vi "SendNoReply.vi"(8 "error in (no error)":errorcluster, 10 "DataIn":string, 11 "index":i32) -> (0 "error out":errorcluster)   [LabVIEW 2019]
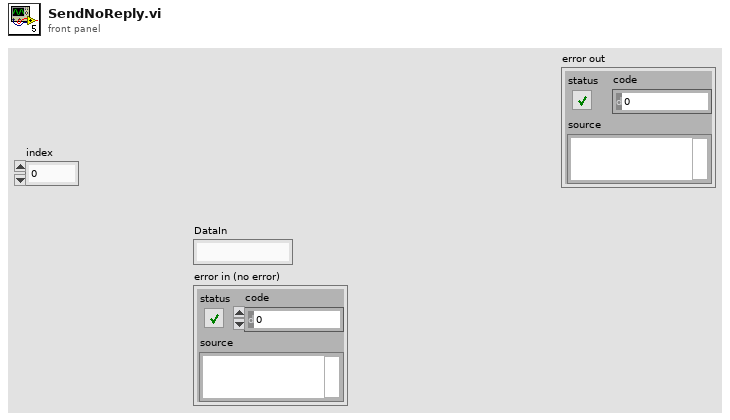
[diagram p1: front panel]
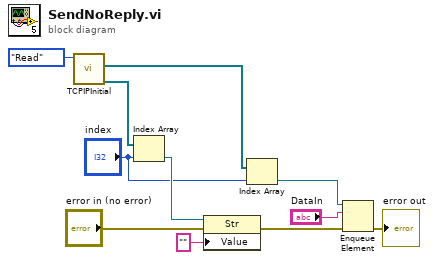
[diagram p0: block diagram]
diagram:
  n1 = call "TCPIPInitial.vi"("Enum"=enum16{"initial", "Read", "release"}."Read") -> ("SN_ReplyRef"=w2:refnum<vi>[], "Sn_cmdQ"=w3:refnum<queue>[])  [unwired: 7 in, 2 out]
  n2 = Index Array(array=w2, index="index") -> (element=w7:refnum<vi>)
  n3 = property class="Str"(reference=w7, error in="error in (no error)", "Value"="") -> (error out=w9:errorcluster)  [unwired: 1 out]
  n4 = Index Array(array=w3, index="index") -> (element=w6:refnum<queue>)
  n5 = Enqueue Element(queue=w6, element="DataIn", error in (no error)=w9) -> (error out=→"error out":errorcluster)  [unwired: 1 in, 2 out]
